vi "ParseVarFile.vi"(8 "data":string) -> (0 "Output varables bytes":i32[](array[numeric]), 1 "Output varables names":string[](array[string]), 2 "Input varables ports":i32[](array[numeric]), 3 "Input varables names":string[](array[string]), 4 "Output varables type":string[](array[string]), 5 "Input varables type":string[](array[string]), 6 "Input varables bytes":i32[](array[numeric]), 7 "Output varables ports":i32[](array[numeric]))   [LabVIEW 2012]
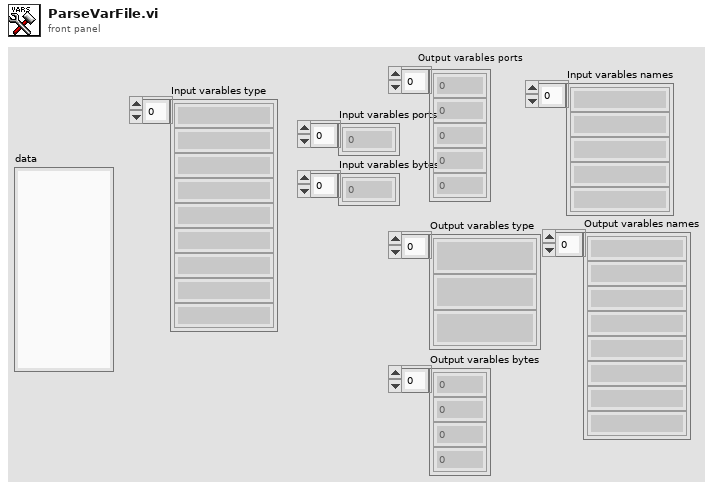
[diagram p1: front panel]
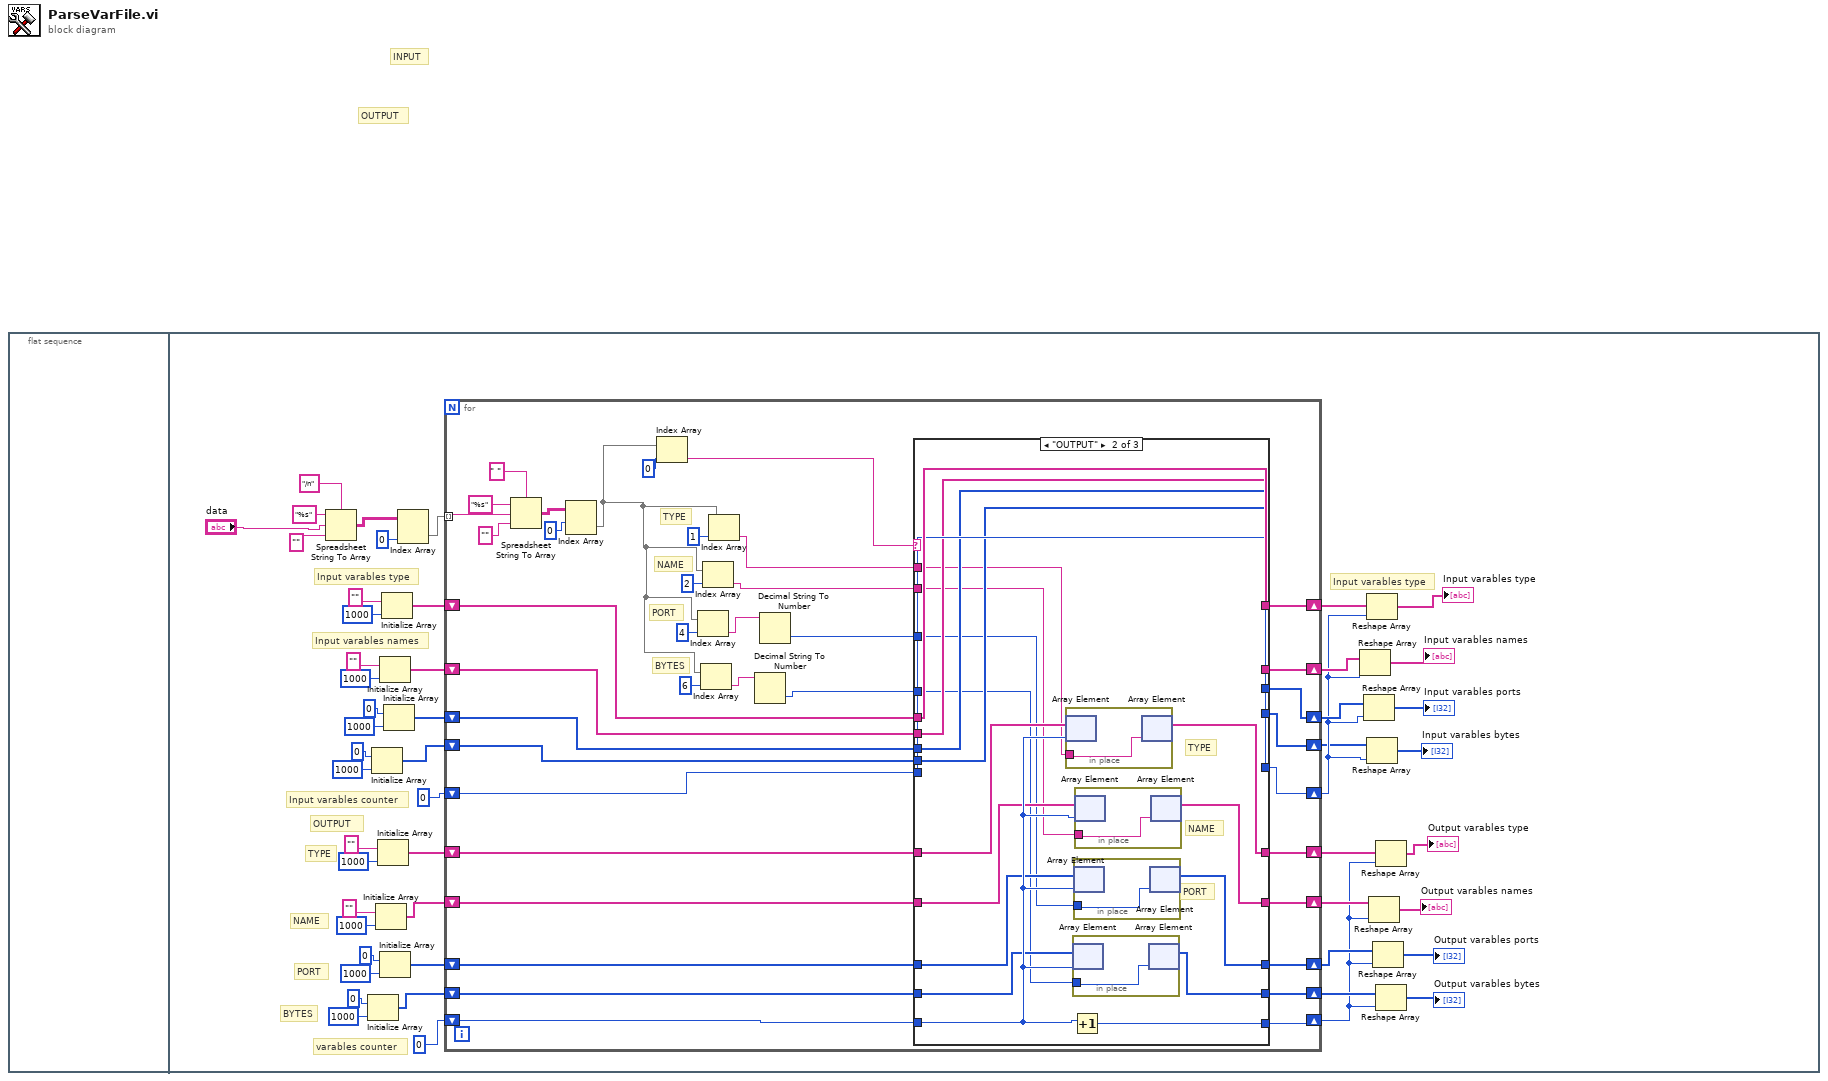
[diagram p0: block diagram]
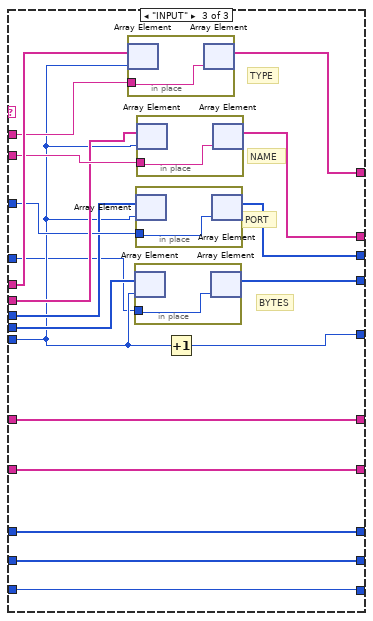
[diagram p3: hidden frame]
diagram:
  # "OUTPUT"
  # "INPUT"
  n1 = flat-sequence {
    frame #0 {
    }
    frame #1 {
      # "NAME"
      # "PORT"
      # "BYTES"
      # "TYPE"
      # "varables counter"
      # "OUTPUT"
      # "Input varables names"
      # "Input varables counter"
      # "Input varables type"
      # "Input varables type"
      n2 = Spreadsheet String To Array(delimiter (Tab)="/n", format string="%s", spreadsheet string="data", array type (2D Dbl)="" ("delimiter (Tab)")) -> (array=w48:string[][])
      n3 = Initialize Array(0 ("dimension size"), 1000 ("dimension size")) -> (w11:i32[])
      n4 = Initialize Array(0 ("dimension size"), 1000 ("dimension size")) -> (w24:i32[])
      n5 = Initialize Array("" ("concatenated string"), 1000 ("dimension size")) -> (w12:string[])
      n6 = Initialize Array("" ("concatenated string"), 1000 ("dimension size")) -> (w13:string[])
      n7 = Initialize Array("" ("concatenated string"), 1000 ("dimension size")) -> (w36:string[])
      n8 = Initialize Array(0 ("dimension size"), 1000 ("dimension size")) -> (w10:i32[])
      n9 = Initialize Array("" ("concatenated string"), 1000 ("dimension size")) -> (w41:string[])
      n10 = Initialize Array(0 ("dimension size"), 1000 ("dimension size")) -> (w33:i32[])
      n11 = Index Array(array=w48, index (col)=0 ("disabled index (col)")) -> (element=w45:string[])  [unwired: 1 in]
      n12 = for {
        tunnel: w45 -> [w85] mode=indexing
        shift-right: [w68] -> w27
        shift-left: 0 ("dimension size") -> [w70]
        shift-right: [w69] -> w40
        shift-left: w41 -> [w71]
        shift-right: [w66] -> w32
        shift-left: w36 -> [w67]
        shift-right: [w64] -> w30
        shift-left: w33 -> [w65]
        shift-right: [w62] -> w23
        shift-left: w24 -> [w63]
        shift-right: [w60] -> w5
        shift-left: 0 ("dimension size") -> [w61]
        shift-right: [w52] -> w9
        shift-left: w13 -> [w59]
        shift-right: [w53] -> w8
        shift-left: w12 -> [w58]
        shift-right: [w54] -> w7
        shift-left: w10 -> [w57]
        shift-right: [w55] -> w6
        shift-left: w11 -> [w56]
        # "BYTES"
        # "PORT"
        # "NAME"
        # "TYPE"
        n13 = Spreadsheet String To Array(delimiter (Tab)=" ", format string="%s", spreadsheet string=w85, array type (2D Dbl)="" ("delimiter (Tab)")) -> (array=w88:string[][])
        n14 = Index Array(array=w88, index (row)=0 ("disabled index (col)")) -> (element=w76:string[])  [unwired: 1 in]
        n15 = Index Array(array=w76, index=0) -> (element=w77:string)
        n16 = Index Array(array=w76, index=4) -> (element=w82:string)
        n17 = Index Array(array=w76, index=6) -> (element=w83:string)
        n18 = Index Array(array=w76, index=2) -> (element=w74:string)
        n19 = Index Array(array=w76, index=1) -> (element=w75:string)
        n20 = Decimal String To Number(string=w83) -> (number=w72:i32)  [unwired: 2 in, 1 out]
        n21 = Decimal String To Number(string=w82) -> (number=w73:i32)  [unwired: 2 in, 1 out]
        n22 = case shown="\"OUTPUT\"" w77 {
          tunnel: w75 -> [_ w109 w141]
          tunnel: w74 -> [_ w108 w139]
          tunnel: w73 -> [_ w105 w135]
          tunnel: w72 -> [_ w102 w130]
          tunnel: w71 -> [w100 w119 w142]
          tunnel: w70 -> [w99 w118 w131]
          tunnel: [w100 w119 w140] -> w69
          tunnel: [w99 w118 w137] -> w68
          tunnel: w67 -> [w98 w117 w138]
          tunnel: [w98 w117 w136] -> w66
          tunnel: w65 -> [w97 w116 w134]
          tunnel: [w97 w116 w133] -> w64
          tunnel: w63 -> [w96 w115 w132]
          tunnel: [w96 w115 w129] -> w62
          tunnel: w61 -> [w95 w111 w128]
          tunnel: [w95 w114 w128] -> w60
          tunnel: w59 -> [w91 w113 w124]
          tunnel: w58 -> [w92 w110 w125]
          tunnel: w57 -> [w93 w106 w126]
          tunnel: w56 -> [w94 w103 w127]
          tunnel: [w94 w101 w127] -> w55
          tunnel: [w93 w104 w126] -> w54
          tunnel: [w92 w107 w125] -> w53
          tunnel: [w91 w112 w124] -> w52
          frame "False", Default {
          }
          frame "OUTPUT" {
            # "PORT"
            # "NAME"
            # "TYPE"
            n23 = in-place {
              in-place-border: w109 -> [w123]
              n24 = in-place-array #1(w113, w111) -> ()  [unwired: 1 out]
              n25 = in-place-array #1(w123) -> (w112:string[])  [unwired: 1 out]
            }
            n26 = Increment(x=w111) -> (x+1=w114:i32)
            n27 = in-place {
              in-place-border: w102 -> [w120]
              n28 = in-place-array #2(w103, w111) -> ()  [unwired: 1 out]
              n29 = in-place-array #2(w120) -> (w101:i32[])  [unwired: 1 out]
            }
            n30 = in-place {
              in-place-border: w105 -> [w121]
              n31 = in-place-array #3(w106, w111) -> ()  [unwired: 1 out]
              n32 = in-place-array #3(w121) -> (w104:i32[])  [unwired: 1 out]
            }
            n33 = in-place {
              in-place-border: w108 -> [w122]
              n34 = in-place-array #4(w110, w111) -> ()  [unwired: 1 out]
              n35 = in-place-array #4(w122) -> (w107:string[])  [unwired: 1 out]
            }
          }
          frame "INPUT" {
            # "BYTES"
            # "PORT"
            # "NAME"
            # "TYPE"
            n36 = in-place {
              in-place-border: w141 -> [w146]
              n37 = in-place-array #5(w142, w131) -> ()  [unwired: 1 out]
              n38 = in-place-array #5(w146) -> (w140:string[])  [unwired: 1 out]
            }
            n39 = in-place {
              in-place-border: w130 -> [w143]
              n40 = in-place-array #6(w132, w131) -> ()  [unwired: 1 out]
              n41 = in-place-array #6(w143) -> (w129:i32[])  [unwired: 1 out]
            }
            n42 = in-place {
              in-place-border: w135 -> [w144]
              n43 = in-place-array #7(w134, w131) -> ()  [unwired: 1 out]
              n44 = in-place-array #7(w144) -> (w133:i32[])  [unwired: 1 out]
            }
            n45 = in-place {
              in-place-border: w139 -> [w145]
              n46 = in-place-array #8(w138, w131) -> ()  [unwired: 1 out]
              n47 = in-place-array #8(w145) -> (w136:string[])  [unwired: 1 out]
            }
            n48 = Increment(x=w131) -> (x+1=w137:i32)
          }
        }
      }
      n49 = Reshape Array(w32, w27) -> (→"Input varables names":string[])
      n50 = Reshape Array(w30, w27) -> (→"Input varables ports":i32[])
      n51 = Reshape Array(w40, w27) -> (→"Input varables type":string[])
      n52 = Reshape Array(w23, w27) -> (→"Input varables bytes":i32[])
      n53 = Reshape Array(w8, w5) -> (→"Output varables names":string[])
      n54 = Reshape Array(w7, w5) -> (→"Output varables ports":i32[])
      n55 = Reshape Array(w9, w5) -> (→"Output varables type":string[])
      n56 = Reshape Array(w6, w5) -> (→"Output varables bytes":i32[])
    }
  }
